vi "calculate_sine_and_advance_phase.vi"(8 "Ramp type":T1, 9 "Cycle parameters in":T4, 10 "Current ramp values":T2, 11 "Cycle counters in":T3) -> (1 "Ramped sine":fxp<+/-,16,12> format="%.28g", 3 "Cycle counters out":T3)   [LabVIEW 2011]
uses:
  typedefs/cycle_parameters_cluster.ctl
  typedefs/cycle_counters_cluster.ctl
  typedefs/current_ramp_values_cluster.ctl
  typedefs/ramp_type_enum.ctl
  <vilib>/rvi/FXPMathLib/FxpSinAndCos/subVIs/nifxpmath_SinAndCos_SimConfig.ctl
  <vilib>/rvi/FXPMathLib/FxpSinAndCos/simVIs/DllFxpSinAndCosTemp_sub.vi
  <vilib>/rvi/FXPMathLib/FxpSinAndCos/XNode/nifxpmath_SinAndCos.xnode
  <vilib>/rvi/FXPMathLib/FxpAdd/XNode/nifxpmath_Add.xnode
  <vilib>/rvi/FXPMathLib/FxpMul/XNode/nifxpmath_Multiplier.xnode
  <vilib>/rvi/FXPMathLib/sim/FxpSim.dll
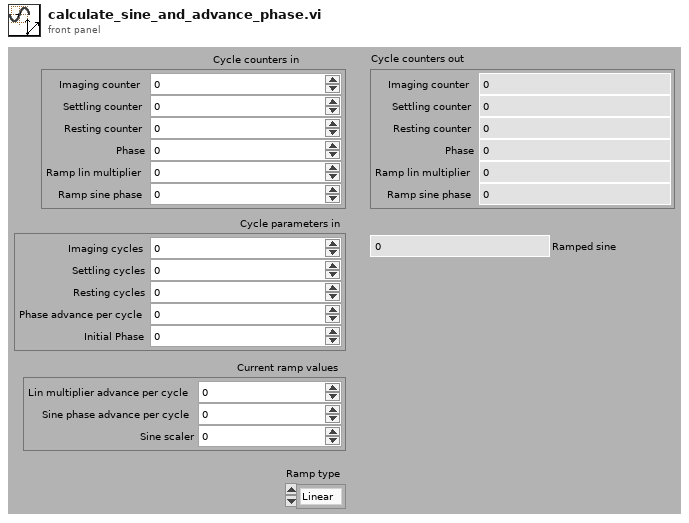
[diagram p1: front panel]
types:
  T1 = typedef "ramp_type_enum.ctl" = enum8{"Linear", "Sine"}
  T2 = typedef "current_ramp_values_cluster.ctl" = cluster{"Lin multiplier advance per cycle":fxp<+/-,32,0>, "Sine phase advance per cycle":fxp<+,32,0>, "Sine scaler":fxp<+,43,12>}
  T3 = typedef "cycle_counters_cluster.ctl" = cluster{"Imaging counter":i32, "Settling counter":i32, "Resting counter":i32, "Phase":fxp<+,32,1>, "Ramp lin multiplier":fxp<+/-,43,12>, "Ramp sine phase":fxp<+,32,1>}
  T4 = typedef "cycle_parameters_cluster.ctl" = cluster{"Imaging cycles":i32, "Settling cycles":i32, "Resting cycles":i32, "Phase advance per cycle":fxp<+,32,0>, "Initial Phase":fxp<+,32,1>}
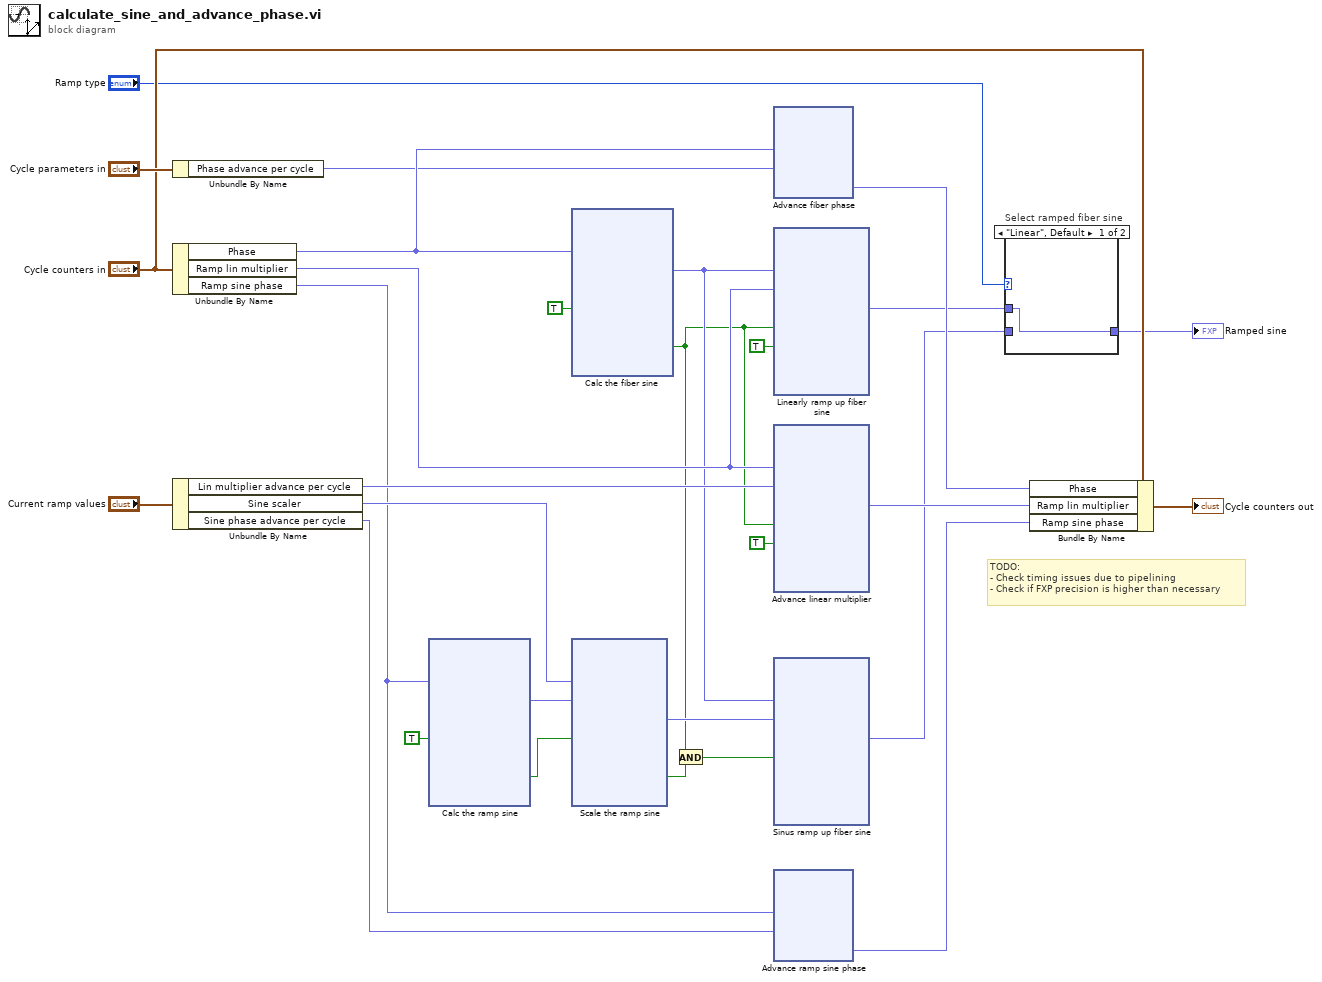
[diagram p0: block diagram]
diagram:
  # "TODO:\n- Check timing issues due to pipelining\n- Check if FXP precision is higher than necessary"
  n1 = Unbundle By Name("Cycle parameters in") -> ("Phase advance per cycle"=w23:fxp<+,32,0>)
  n2 = Unbundle By Name("Cycle counters in") -> ("Phase"=w25:fxp<+,32,1>, "Ramp lin multiplier"=w26:fxp<+/-,43,12>, "Ramp sine phase"=w1:fxp<+,32,1>)
  n3 = Unbundle By Name("Current ramp values") -> ("Lin multiplier advance per cycle"=w18:fxp<+/-,32,0>, "Sine scaler"=w15:fxp<+,43,12>, "Sine phase advance per cycle"=w7:fxp<+,32,0>)
  n4 = xnode "Calc the ramp sine"("x (pi)"=w1, "input valid"=TRUE) -> ("sin(x)"=w14:fxp<+/-,32,2>, "output valid"=w13:bool)  [unwired: 1 in, 2 out]
  n5 = xnode "Calc the fiber sine"("x (pi)"=w25, "input valid"=TRUE) -> ("sin(x)"=w12:fxp<+/-,32,2>, "output valid"=w9:bool)  [unwired: 1 in, 2 out]
  n6 = xnode "Scale the ramp sine"("x"=w15, "y"=w14, "input valid"=w13) -> ("x*y"=w11:fxp<+/-,43,12>, "output valid"=w10:bool)  [unwired: 1 in, 1 out]
  n7 = And(x=w9, y=w10) -> (x .and. y?=w8:bool)
  n8 = xnode "Advance fiber phase"("x"=w25, "y"=w23) -> ("x+y"=w21:fxp<+,32,1>)
  n9 = xnode "Linearly ramp up fiber sine"("x"=w12, "y"=w26, "input valid"=w9, "ready for output (T)"=TRUE) -> ("x*y"=w4:fxp<+/-,16,12>)  [unwired: 2 out]
  n10 = xnode "Advance linear multiplier"("x"=w26, "y"=w18, "input valid"=w9, "ready for output (T)"=TRUE) -> ("x+y"=w20:fxp<+/-,43,12>)  [unwired: 2 out]
  n11 = xnode "Sinus ramp up fiber sine"("x"=w12, "y"=w11, "input valid"=w8) -> ("x*y"=w3:fxp<+/-,16,12>)  [unwired: 1 in, 2 out]
  n12 = xnode "Advance ramp sine phase"("x"=w1, "y"=w7) -> ("x+y"=w6:fxp<+,32,1>)
  n13 = case "Select ramped fiber sine" shown="\"Linear\", Default" "Ramp type" {
    tunnel: w4 -> [w30 _]
    tunnel: w3 -> [_ w31]
    tunnel: [w30 w31] -> w2
    frame "Linear", Default {
    }
    frame "Sine" {
    }
  }
  "Ramped sine" <- w2
  n14 = Bundle By Name(cluster="Cycle counters in", "Phase"=w21, "Ramp lin multiplier"=w20, "Ramp sine phase"=w6) -> (→"Cycle counters out":T3)
